vi "Identify Delay Generator.vi"(8 "error in":errorcluster, 11 "VISA resource name":refnum<visa-resource-name>) -> (0 "error out":errorcluster, 1 "Delay Generator Driver.lvclass":refnum<class "Delay Generator Driver.lvclass">, 2 "Status byte":i32 format="%b", 3 "VISA resource name out":refnum<visa-resource-name>)   [LabVIEW 2020]
uses:
  Delay Generator Driver/Delay Generator Driver.lvclass
  C:/GitHub/NHMFL_Core/Libraries/Instruments/VISA Instrument/VISA Instrument.lvclass
  DG635/DG635 Driver/DG635 Driver.lvclass
  C:/GitHub/NHMFL_Core/Libraries/Instruments/SRS/Delay Generator/Delay Generator Driver/Delay Generator Driver.lvclass
  DG535/DG535 Driver/DG535 Driver.lvclass
  VISA Instrument/VISA Instrument.lvclass/VISA Instrument.ctl
  VISA Instrument/Write VISA resource.vi
panel:
  out "data string out":string
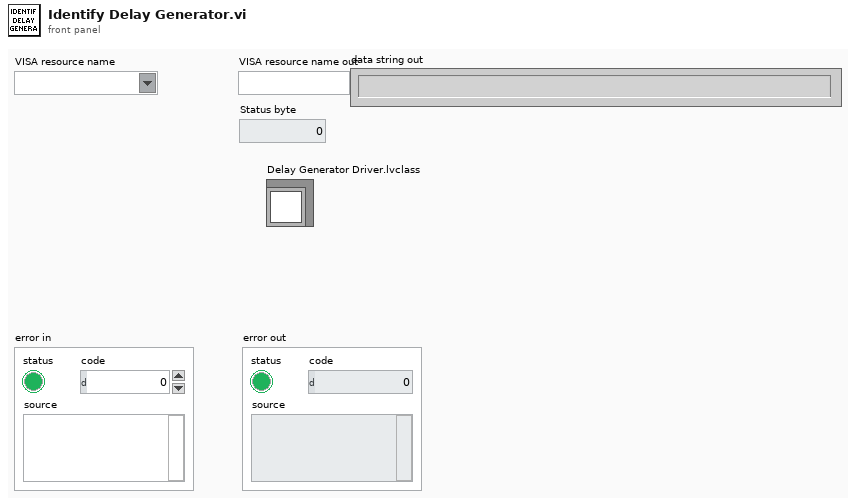
[diagram p1: front panel]
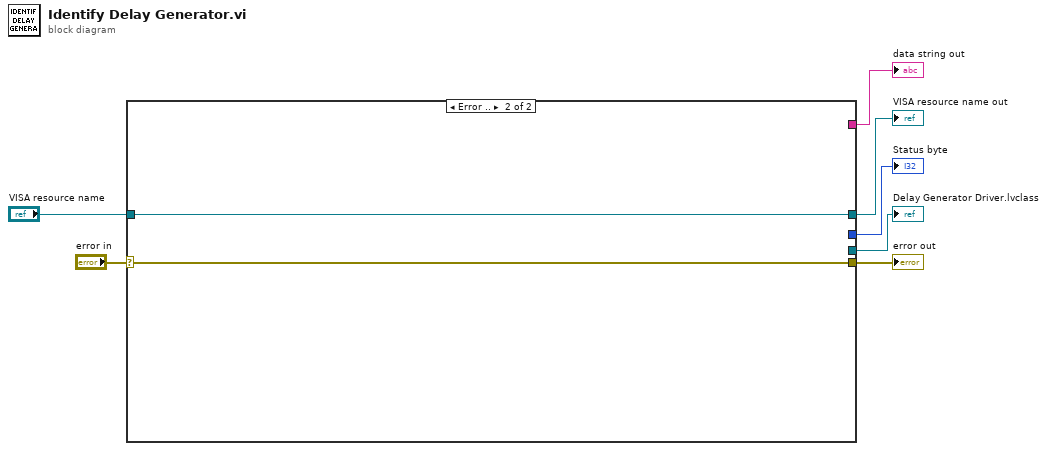
[diagram p0: block diagram]
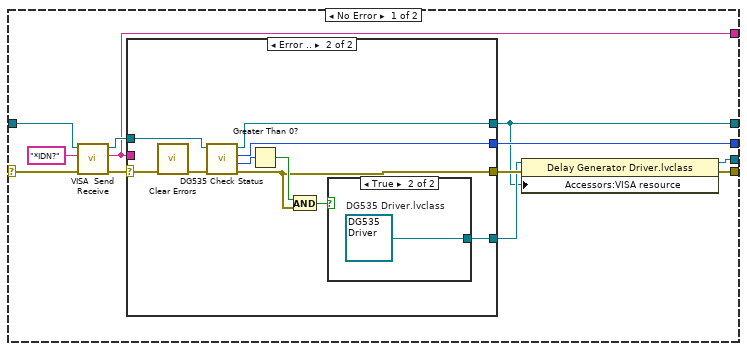
[diagram p2: hidden frame]
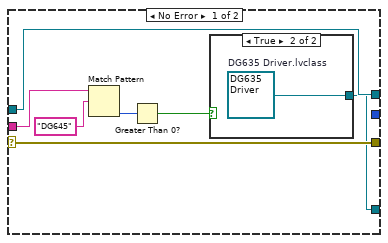
[diagram p3: hidden frame]
diagram:
  n1 = case shown="Error .." "error in" {
    selector: "error in" -> [w8 w40]
    tunnel: "VISA resource name" -> [w18 w39]
    tunnel: [w14 _] -> w6
    tunnel: [w13 _] -> w5
    tunnel: [w12 w40] -> w4
    tunnel: [w10 _] -> w3
    tunnel: [w9 w39] -> w2
    frame No Error {
      n2 = call "VISA  Send Receive.vi"("error in (no error)"=w8, "data string in"="*IDN?", "VISA Resource Name"=w18) -> ("error out"=w17:errorcluster, "data string out"=w13:string, "VISA Resource Name Out"=w16:refnum<visa-resource-name>)  [unwired: 6 in]
      n3 = case shown="Error .." w17 {
        selector: w17 -> [w26 w37]
        tunnel: w16 -> [w25 w35]
        tunnel: [w20 w31] -> w11
        tunnel: [w26 w30] -> w15
        tunnel: [_ w29] -> w14
        tunnel: [w25 w28] -> w9
        tunnel: w13 -> [w24 _]
        frame No Error {
          n4 = Match Pattern(string=w24, regular expression="DG645") -> (offset past match=w22:i32)  [unwired: 1 in, 3 out]
          n5 = Greater Than 0?(x=w22) -> (x > 0?=w21:bool)
          n6 = case shown="True" w21 {
            tunnel: [_ w27] -> w20
            frame False {
            }
            frame True {
              w27 = refnum<class "DG635 Driver.lvclass"> refnum  # DG635 Driver.lvclass
            }
          }
        }
        frame Error {
          n7 = call <vilib>:"Clear Errors.vi"("error in (no error)"=w37) -> ("error out"=w36:errorcluster)  [unwired: 5 in, 1 out]
          n8 = call "DG535 Check Status.vi"("error in"=w36, "VISA resource name"=w35) -> ("error out"=w30:errorcluster, "offset past number"=w34:i32, "Status byte"=w29:i32, "VISA resource name out"=w28:refnum<visa-resource-name>)  [unwired: 6 in]
          n9 = Greater Than 0?(x=w34) -> (x > 0?=w33:bool)
          n10 = And(x=w33, y=w30) -> (x .and. y?=w32:bool)
          n11 = case shown="True" w32 {
            tunnel: [_ w38] -> w31
            frame False {
            }
            frame True {
              w38 = refnum<class "DG535 Driver.lvclass"> refnum  # DG535 Driver.lvclass
            }
          }
        }
      }
      n12 = property class="Delay Generator Driver.lvclass"(reference=w11, error in=w15, "Accessors:VISA resource"=w9) -> (reference out=w10:refnum<class "Delay Generator Driver.lvclass">, error out=w12:errorcluster)
    }
    frame Error {
    }
  }
  "error out" <- w4
  "Status byte" <- w6
  "Delay Generator Driver.lvclass" <- w3
  "data string out" <- w5
  "VISA resource name out" <- w2
